vi "ButtonPickupRecycleBinAuto.vi"(11 "Buttons":bool[](array[boolean])) -> (3 "Boolean":bool)   [LabVIEW 2014]
uses:
  LowerLiftAndOpenArms.ctl
  Gantry/GantryGlobals.vi
  ToteCount.vi
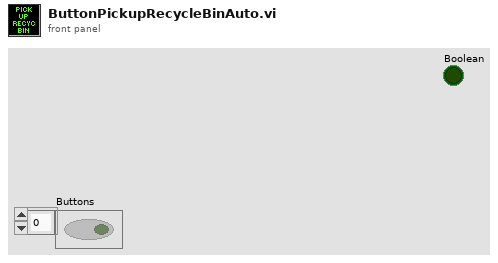
[diagram p1: front panel]
types:
  T1 = typedef "LowerLiftAndOpenArms.ctl" = enum16{"WaitingForInput", "LowerLift", "OpenArms", "LowerLiftMore", "CloseArms", "RaiseLift", "StopArms"}
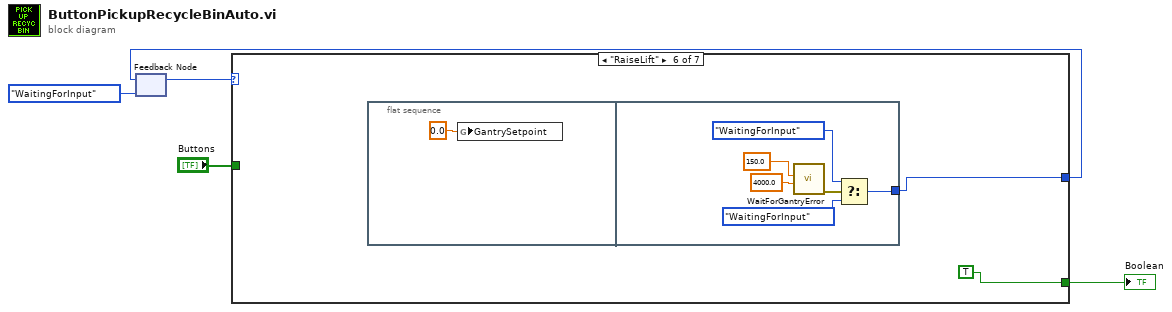
[diagram p0: block diagram]
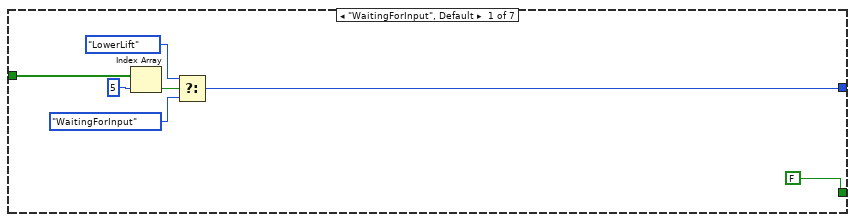
[diagram p2: hidden frame]
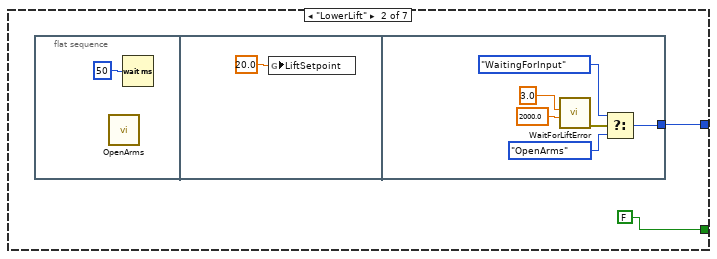
[diagram p3: hidden frame]
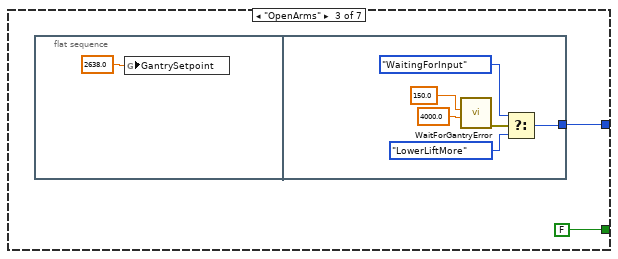
[diagram p4: hidden frame]
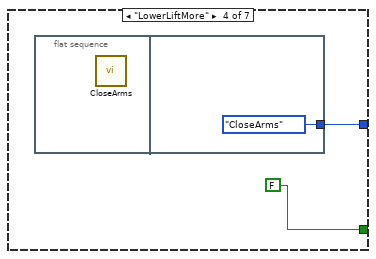
[diagram p5: hidden frame]
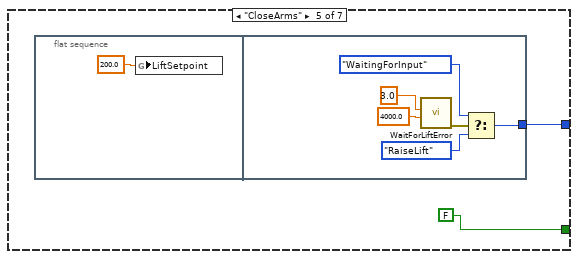
[diagram p6: hidden frame]
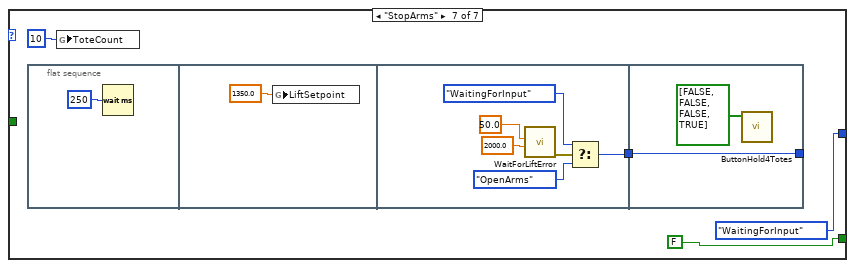
[diagram p7: hidden frame]
diagram:
  n1 = feedback #1(LowerLiftAndOpenArms."WaitingForInput" ("LowerAndOpen")) -> (w4:T1)
  n2 = case shown="\"RaiseLift\"" w4 {
    tunnel: [w7 w14 w24 w33 w36 w45 LowerLiftAndOpenArms."WaitingForInput" ("LowerAndOpen")] -> w5
    tunnel: "Buttons" -> [w11 _ _ _ _ _ _]
    tunnel: [FALSE FALSE FALSE FALSE FALSE TRUE FALSE] -> w1
    frame "WaitingForInput", Default {
      n3 = Index Array(array=w11, index=5) -> (element=w8:bool)
      n4 = Select(t=LowerLiftAndOpenArms."LowerLift" ("LowerAndOpen"), s=w8, f=LowerLiftAndOpenArms."WaitingForInput" ("LowerAndOpen")) -> (s? t:f=w7:T1)
    }
    frame "LowerLift" {
      n5 = flat-sequence {
        tunnel: [w17] -> w14
        frame #0 {
          n6 = call "OpenArms.vi"() -> ()  [unwired: 12 in]
          n7 = Wait (ms)(milliseconds to wait=u32 50) -> ()  [unwired: 1 out]
        }
        frame #1 {
          n8 = global write "GantryGlobals.vi" "LiftSetpoint"(20.0 ("LiftSetpoint")) -> ()
        }
        frame #2 {
          n9 = call "WaitForLiftError.vi"("Timeout (ms)"=2000.0, "AllowedError"=3.0) -> ("error out"=w20:errorcluster)  [unwired: 9 in]
          n10 = Select(t=LowerLiftAndOpenArms."WaitingForInput" ("LowerAndOpen"), s=w20, f=LowerLiftAndOpenArms."OpenArms" ("LowerAndOpen")) -> (s? t:f=w17:T1)
        }
      }
    }
    frame "OpenArms" {
      n11 = flat-sequence {
        tunnel: [w26] -> w24
        frame #0 {
          n12 = global write "GantryGlobals.vi" "GantrySetpoint"(2638.0 ("GantrySetpoint")) -> ()
        }
        frame #1 {
          n13 = call "WaitForGantryError.vi"("Timeout (ms)"=4000.0, "AllowedError"=150.0) -> ("error out"=w28:errorcluster)  [unwired: 9 in]
          n14 = Select(t=LowerLiftAndOpenArms."WaitingForInput", s=w28, f=LowerLiftAndOpenArms."LowerLiftMore" ("LowerAndOpen")) -> (s? t:f=w26:T1)
        }
      }
    }
    frame "LowerLiftMore" {
      n15 = flat-sequence {
        tunnel: [LowerLiftAndOpenArms."CloseArms" ("LowerAndOpen")] -> w33
        frame #0 {
          n16 = call "CloseArms.vi"() -> ()  [unwired: 12 in]
        }
        frame #1 {
        }
      }
    }
    frame "CloseArms" {
      n17 = flat-sequence {
        tunnel: [w38] -> w36
        frame #0 {
          n18 = global write "GantryGlobals.vi" "LiftSetpoint"(200.0 ("LiftSetpoint")) -> ()
        }
        frame #1 {
          n19 = call "WaitForLiftError.vi"("Timeout (ms)"=4000.0, "AllowedError"=3.0) -> ("error out"=w41:errorcluster)  [unwired: 9 in]
          n20 = Select(t=LowerLiftAndOpenArms."WaitingForInput" ("LowerAndOpen"), s=w41, f=LowerLiftAndOpenArms."RaiseLift" ("LowerAndOpen")) -> (s? t:f=w38:T1)
        }
      }
    }
    frame "RaiseLift" {
      n21 = flat-sequence {
        tunnel: [w47] -> w45
        frame #0 {
          n22 = global write "GantryGlobals.vi" "GantrySetpoint"(0.0 ("GantrySetpoint")) -> ()
        }
        frame #1 {
          n23 = call "WaitForGantryError.vi"("Timeout (ms)"=4000.0, "AllowedError"=150.0) -> ("error out"=w49:errorcluster)  [unwired: 9 in]
          n24 = Select(t=LowerLiftAndOpenArms."WaitingForInput", s=w49, f=LowerLiftAndOpenArms."WaitingForInput" ("LowerAndOpen")) -> (s? t:f=w47:T1)
        }
      }
    }
    frame "StopArms" {
      n25 = flat-sequence {
        tunnel: [w59] -> w54
        tunnel: [w66] -> _
        tunnel: w54 -> [w66]
        frame #0 {
          n26 = Wait (ms)(milliseconds to wait=u32 250) -> ()  [unwired: 1 out]
        }
        frame #1 {
          n27 = global write "GantryGlobals.vi" "LiftSetpoint"(1350.0 ("LiftSetpoint")) -> ()
        }
        frame #2 {
          n28 = call "WaitForLiftError.vi"("Timeout (ms)"=2000.0, "AllowedError"=50.0) -> ("error out"=w62:errorcluster)  [unwired: 9 in]
          n29 = Select(t=LowerLiftAndOpenArms."WaitingForInput" ("LowerAndOpen"), s=w62, f=LowerLiftAndOpenArms."OpenArms" ("LowerAndOpen")) -> (s? t:f=w59:T1)
        }
        frame #3 {
          n30 = call "ButtonHold4Totes.vi"("Buttons"=bool[] [FALSE, FALSE, FALSE, TRUE]) -> ()  [unwired: 10 in, 1 out]
        }
      }
      n31 = global write "ToteCount.vi" "ToteCount"(10 ("ToteCount")) -> ()
    }
  }
  "Boolean" <- w1
  n32 = feedback-in #1(w5) -> ()
